vi "MegaAnalysis5.vi"() -> ()   [LabVIEW 2016] (continued)
                            tunnel: w2920 -> [_ _ w2954 w2987]
                            tunnel: [w2924 w2925 w2937 w2970] -> w2919
                            tunnel: [w2924 w2925 w2931 w2964] -> w2918
                            tunnel: [w2924 w2925 w2936 w2969] -> w2917
                            tunnel: [w2924 w2925 w2926 w2959] -> w2916
                            frame 0, Default {
                              w2924 = 0
                            }
                            frame 1 {
                              w2925 = 0
                            }
                            frame 2 {
                              n1178 = call "readbinary.vi"(7:w2956, "base path"=w2954, "file index"=w2955, "data column"="bclr") -> ("data"=w2947:ext[])  [unwired: 7 out]
                              n1179 = call "readbinary.vi"(7:w2956, "base path"=w2954, "file index"=w2955, "data column"="bclf") -> ("data"=w2944:ext[])  [unwired: 7 out]
                              n1180 = Array Max & Min(array=w2944) -> (max value=w2952:ext, min value=w2950:ext)  [unwired: 2 out]
                              n1181 = Array Max & Min(array=w2947) -> (max value=w2953:ext, min value=w2951:ext)  [unwired: 2 out]
                              n1182 = Max & Min(x=w2953, y=w2952) -> (min(x,y)=w2943:ext)  [unwired: 1 out]
                              n1183 = Max & Min(x=w2951, y=w2950) -> (max(x,y)=w2942:ext)  [unwired: 1 out]
                              n1184 = Subtract(x=w2944, y=w2943) -> (x-y=w2941:ext[])
                              n1185 = Subtract(x=w2944, y=w2942) -> (x-y=w2940:ext[])
                              n1186 = Subtract(x=w2947, y=w2943) -> (x-y=w2949:ext[])
                              n1187 = Subtract(x=w2947, y=w2942) -> (x-y=w2946:ext[])
                              n1188 = Absolute Value(x=w2946) -> (abs(x)=w2945:ext[])
                              n1189 = Absolute Value(x=w2941) -> (abs(x)=w2939:ext[])
                              n1190 = Absolute Value(x=w2949) -> (abs(x)=w2948:ext[])
                              n1191 = Absolute Value(x=w2940) -> (abs(x)=w2938:ext[])
                              n1192 = Array Max & Min(array=w2945) -> (min index (indices)=w2934:i32)  [unwired: 3 out]
                              n1193 = Array Max & Min(array=w2948) -> (min index (indices)=w2935:i32)  [unwired: 3 out]
                              n1194 = Array Max & Min(array=w2938) -> (min index (indices)=w2929:i32)  [unwired: 3 out]
                              n1195 = Array Max & Min(array=w2939) -> (min index (indices)=w2930:i32)  [unwired: 3 out]
                              n1196 = Subtract(x=w2935, y=w2934) -> (x-y=w2933:i32)
                              n1197 = Absolute Value(x=w2933) -> (abs(x)=w2932:i32)
                              n1198 = Max & Min(x=w2930, y=w2929) -> (min(x,y)=w2936:i32)  [unwired: 1 out]
                              n1199 = Max & Min(x=w2935, y=w2934) -> (min(x,y)=w2937:i32)  [unwired: 1 out]
                              n1200 = Subtract(x=w2930, y=w2929) -> (x-y=w2928:i32)
                              n1201 = Absolute Value(x=w2928) -> (abs(x)=w2927:i32)
                              n1202 = Increment(x=w2927) -> (x+1=w2926:i32)
                              n1203 = Increment(x=w2932) -> (x+1=w2931:i32)
                            }
                            frame 3 {
                              n1204 = call "readbinary.vi"(7:w2989, "base path"=w2987, "file index"=w2988, "data column"="bclr") -> ("data"=w2980:ext[])  [unwired: 7 out]
                              n1205 = call "readbinary.vi"(7:w2989, "base path"=w2987, "file index"=w2988, "data column"="bclf") -> ("data"=w2977:ext[])  [unwired: 7 out]
                              n1206 = Array Max & Min(array=w2977) -> (max value=w2985:ext, min value=w2983:ext)  [unwired: 2 out]
                              n1207 = Array Max & Min(array=w2980) -> (max value=w2986:ext, min value=w2984:ext)  [unwired: 2 out]
                              n1208 = Max & Min(x=w2986, y=w2985) -> (min(x,y)=w2976:ext)  [unwired: 1 out]
                              n1209 = Max & Min(x=w2984, y=w2983) -> (max(x,y)=w2975:ext)  [unwired: 1 out]
                              n1210 = Subtract(x=w2977, y=w2976) -> (x-y=w2974:ext[])
                              n1211 = Subtract(x=w2977, y=w2975) -> (x-y=w2973:ext[])
                              n1212 = Subtract(x=w2980, y=w2976) -> (x-y=w2982:ext[])
                              n1213 = Subtract(x=w2980, y=w2975) -> (x-y=w2979:ext[])
                              n1214 = Absolute Value(x=w2979) -> (abs(x)=w2978:ext[])
                              n1215 = Absolute Value(x=w2974) -> (abs(x)=w2972:ext[])
                              n1216 = Absolute Value(x=w2982) -> (abs(x)=w2981:ext[])
                              n1217 = Absolute Value(x=w2973) -> (abs(x)=w2971:ext[])
                              n1218 = Array Max & Min(array=w2978) -> (min index (indices)=w2967:i32)  [unwired: 3 out]
                              n1219 = Array Max & Min(array=w2981) -> (min index (indices)=w2968:i32)  [unwired: 3 out]
                              n1220 = Array Max & Min(array=w2971) -> (min index (indices)=w2962:i32)  [unwired: 3 out]
                              n1221 = Array Max & Min(array=w2972) -> (min index (indices)=w2963:i32)  [unwired: 3 out]
                              n1222 = Subtract(x=w2968, y=w2967) -> (x-y=w2966:i32)
                              n1223 = Absolute Value(x=w2966) -> (abs(x)=w2965:i32)
                              n1224 = Max & Min(x=w2963, y=w2962) -> (min(x,y)=w2969:i32)  [unwired: 1 out]
                              n1225 = Max & Min(x=w2968, y=w2967) -> (min(x,y)=w2970:i32)  [unwired: 1 out]
                              n1226 = Subtract(x=w2963, y=w2962) -> (x-y=w2961:i32)
                              n1227 = Absolute Value(x=w2961) -> (abs(x)=w2960:i32)
                              n1228 = Increment(x=w2960) -> (x+1=w2959:i32)
                              n1229 = Increment(x=w2965) -> (x+1=w2964:i32)
                            }
                          }
                        }
                        frame #9 {
                          n1230 = case shown="0, Default" w3001 {
                            tunnel: w3000 -> [_ _ w3010 w3032]
                            tunnel: w2999 -> [_ _ w3009 w3031]
                            tunnel: w2998 -> [_ _ w3008 w3030]
                            tunnel: w2997 -> [_ _ w3007 w3029]
                            tunnel: w2996 -> [_ _ w3006 w3028]
                            tunnel: w2995 -> [_ _ w3005 w3027]
                            tunnel: w2994 -> [_ _ w3004 w3026]
                            tunnel: w2993 -> [_ _ w3003 w3025]
                            tunnel: w2992 -> [_ _ w3002 w3024]
                            frame 0, Default {
                            }
                            frame 1 {
                            }
                            frame 2 {
                              n1231 = for {
                                tunnel: w3010 -> [w3013] mode=indexing
                                tunnel: w3009 -> [w3014] mode=indexing
                                tunnel: w3008 -> [w3012]
                                tunnel: w3007 -> [w3011]
                                tunnel: w3006 -> [w3015]
                                tunnel: w3005 -> [w3021]
                                tunnel: w3004 -> [w3020]
                                tunnel: w3003 -> [w3019]
                                tunnel: w3002 -> [w3018]
                                n1232 = call "readbinary.vi"(7:w3015, "base path"=w3011, "file index"=w3012, "data column"=w3013) -> ("data"=w3023:ext[])  [unwired: 7 out]
                                n1233 = call "readbinary.vi"(7:w3015, "base path"=w3011, "file index"=w3012, "data column"=w3014) -> ("data"=w3022:ext[])  [unwired: 7 out]
                                n1234 = Array Subset(array=w3022, index=w3020, length=w3018) -> (w3016:ext[])
                                n1235 = Array Subset(array=w3023, index=w3021, length=w3019) -> (w3017:ext[])
                                n1236 = call "writebinary.vi"(7:w3015, "base path"=w3011, "file index"=w3012, "data column"=w3014, "data"=w3016) -> ()  [unwired: 7 out]
                                n1237 = call "writebinary.vi"(7:w3015, "base path"=w3011, "file index"=w3012, "data column"=w3013, "data"=w3017) -> ()  [unwired: 7 out]
                              }
                            }
                            frame 3 {
                              n1238 = for {
                                tunnel: w3032 -> [w3035] mode=indexing
                                tunnel: w3031 -> [w3036] mode=indexing
                                tunnel: w3030 -> [w3034]
                                tunnel: w3029 -> [w3033]
                                tunnel: w3028 -> [w3037]
                                tunnel: w3027 -> [w3043]
                                tunnel: w3026 -> [w3042]
                                tunnel: w3025 -> [w3041]
                                tunnel: w3024 -> [w3040]
                                n1239 = call "readbinary.vi"(7:w3037, "base path"=w3033, "file index"=w3034, "data column"=w3035) -> ("data"=w3045:ext[])  [unwired: 7 out]
                                n1240 = call "readbinary.vi"(7:w3037, "base path"=w3033, "file index"=w3034, "data column"=w3036) -> ("data"=w3044:ext[])  [unwired: 7 out]
                                n1241 = Array Subset(array=w3044, index=w3042, length=w3040) -> (w3038:ext[])
                                n1242 = Array Subset(array=w3045, index=w3043, length=w3041) -> (w3039:ext[])
                                n1243 = call "writebinary.vi"(7:w3037, "base path"=w3033, "file index"=w3034, "data column"=w3036, "data"=w3038) -> ()  [unwired: 7 out]
                                n1244 = call "writebinary.vi"(7:w3037, "base path"=w3033, "file index"=w3034, "data column"=w3035, "data"=w3039) -> ()  [unwired: 7 out]
                              }
                            }
                          }
                        }
                      }
                    }
                    n1245 = Boolean To (0,1)(Boolean=w2674) -> (0, 1=w2673:i16[])
                    n1246 = Add Array Elements(numeric array=w2673) -> (sum=w2672:i16)
                    n1247 = Not Equal To 0?(x=w2672) -> (x != 0?=w2669:bool)
                    n1248 = And(x=w2669, y=w2668) -> (x .and. y?=→"dddd":bool)
                  }
                }
              }
            }
          }
          frame #7 {
            n1249 = case shown="True" w3051 {
              tunnel: w3050 -> [_ w3071]
              tunnel: w3049 -> [_ w3072]
              tunnel: w3048 -> [_ w3073]
              tunnel: [w3056 w3062] -> w3047
              tunnel: w3046 -> [_ w3059]
              frame False {
                w3057 = dbl[] [] ("Array 11")
                n1250 = Bundle("Array 11"=w3057, "Array 11"=w3057) -> (w3055:cluster{"Array 11":dbl[], "Array 11":dbl[]})  [unwired: 1 out]
                n1251 = Build Array(w3055) -> (w3056:cluster{"Array 11":dbl[], "Array 11":dbl[]}[])
              }
              frame True {
                n1252 = Build Path(base path=w3071, name or relative path="files2") -> (appended path=w3069:path)
                n1253 = call-poly <vilib>:"Read From Spreadsheet File.vi"("file path (dialog if empty)"=w3069) -> ("first row"=w3060:string[])  [unwired: 3 in, 7 out]
                n1254 = for {
                  tunnel: w3071 -> [w3102]
                  tunnel: w3073 -> [w3106]
                  tunnel: w3072 -> [w3103]
                  tunnel: w3060 -> [_] mode=indexing
                  tunnel: [w3094] -> w3068 mode=indexing
                  tunnel: [w3093] -> w3067 mode=indexing
                  tunnel: w3059 -> [w3092]
                  i -> [w3101]
                  n1255 = Index Array(array=w3106, index="y axis") -> (element=w3099:string)
                  n1256 = Index Array(array=w3103, index="x axis") -> (element=w3098:string)
                  n1257 = Index Array(array=w3106, index="x axis") -> (element=w3097:string)
                  n1258 = Index Array(array=w3103, index="y axis") -> (element=w3100:string)
                  n1259 = call "readbinary.vi"(7:w3092, "base path"=w3102, "file index"=w3101, "data column"=w3098) -> ("data"=w3095:ext[])  [unwired: 7 out]
                  n1260 = call "readbinary.vi"(7:w3092, "base path"=w3102, "file index"=w3101, "data column"=w3097) -> ("data"=w3108:ext[])  [unwired: 7 out]
                  n1261 = call "readbinary.vi"(7:w3092, "base path"=w3102, "file index"=w3101, "data column"=w3099) -> ("data"=w3107:ext[])  [unwired: 7 out]
                  n1262 = call "readbinary.vi"(7:w3092, "base path"=w3102, "file index"=w3101, "data column"=w3100) -> ("data"=w3096:ext[])  [unwired: 7 out]
                  n1263 = Bundle("data"=w3095, "data"=w3096) -> (w3094:cluster{"data":ext[], "data":ext[]})  [unwired: 1 out]
                  n1264 = Bundle("data"=w3108, "data"=w3107) -> (w3093:cluster{"data":ext[], "data":ext[]})  [unwired: 1 out]
                }
                n1265 = Array Size(array=w3060) -> (size(s)=w3066:i32)
                n1266 = Multiply(x=w3066, y=2) -> (x*y=w3064:i32)
                n1267 = global write "status.vi" "String"("plotting selected data") -> ()
                n1268 = for {
                  N: w3064 -> [_]
                  tunnel: w3068 -> [w3076]
                  tunnel: w3067 -> [w3077]
                  shift-right: [w3080] -> _
                  shift-left: 0 -> [w3074]
                  tunnel: [w3075] -> w3062 mode=indexing
                  tunnel: [w3074] -> w3061 mode=indexing
                  i -> [w3078]
                  n1269 = case shown="0, Default" w3074 {
                    tunnel: w3078 -> [w3084 w3091]
                    tunnel: w3077 -> [w3083 _]
                    tunnel: [w3081 w3087] -> w3075
                    tunnel: w3076 -> [_ w3088]
                    frame 0, Default {
                      n1270 = Divide(x=w3084, y=2) -> (x/y=w3082:dbl)
                      n1271 = Index Array(array=w3083, index=w3082) -> (element=w3081:cluster{"data":ext[], "data":ext[]})
                    }
                    frame 1 {
                      n1272 = Decrement(x=w3091) -> (x-1=w3090:i32)
                      n1273 = Divide(x=w3090, y=2) -> (x/y=w3089:dbl)
                      n1274 = Index Array(array=w3088, index=w3089) -> (element=w3087:cluster{"data":ext[], "data":ext[]})
                    }
                  }
                  n1275 = Subtract(x=1, y=w3074) -> (x-y=w3080:i32)
                }
                n1276 = for {
                  tunnel: w3061 -> [_] mode=indexing
                }
              }
            }
            "?" <- w3047
            n1277 = while {
              stop <- w3053 stop-if-true
              n1278 = Not(x="?") -> (.not. x?=w3053:bool)
              n1279 = Wait (ms)(milliseconds to wait=1000) -> ()  [unwired: 1 out]
            }
          }
          frame #8 {
            n1280 = Build Path(base path=w3112, name or relative path="files2") -> (appended path=w3120:path)
            n1281 = Build Path(base path=w3112, name or relative path="paths2") -> (appended path=w3117:path)
            n1282 = call-poly <vilib>:"Read From Spreadsheet File.vi"("file path (dialog if empty)"=w3120) -> ("first row"=w3119:string[])  [unwired: 3 in, 7 out]
            n1283 = call-poly <vilib>:"Read From Spreadsheet File.vi"("file path (dialog if empty)"=w3117) -> ("first row"=w3115:string[])  [unwired: 3 in, 7 out]
            n1284 = String To Path(string=w3115) -> (path=w3116:path[])
            n1285 = case shown="True" w3123 {
              tunnel: w3119 -> [_ w3135]
              tunnel: w3116 -> [_ w3134]
              tunnel: w3122 -> [_ w3133]
              tunnel: w3112 -> [_ w3126]
              tunnel: "file format" -> [_ w3132]
              tunnel: w3113 -> [_ w3131]
              tunnel: w3111 -> [_ w3129]
              tunnel: w3110 -> [w3124 w3128]
              tunnel: [w3124 w3127] -> w3109
              frame False {
              }
              frame True {
                n1286 = for {
                  tunnel: w3135 -> [w3156] mode=indexing
                  tunnel: w3134 -> [w3154] mode=indexing
                  tunnel: "append name" -> [w3155]
                  tunnel: w3133 -> [w3150]
                  tunnel: w3126 -> [w3148]
                  tunnel: w3132 -> [w3145]
                  tunnel: w3131 -> [w3144]
                  tunnel: w3129 -> [w3142]
                  shift-right: [w3140] -> w3127
                  shift-left: w3128 -> [w3139]
                  tunnel: w3126 -> [w3137]
                  i -> [w3149]
                  n1287 = call "filecount.vi"("Path"=w3137) -> ("file count string"=w3136:string)  [unwired: 10 out]
                  n1288 = Concatenate Strings("mega", w3136, w3156, w3155) -> (w3153:string)
                  n1289 = Build Path(base path=w3154, name or relative path=w3153) -> (appended path=w3138:path)
                  n1290 = Build Array (concatenate)(w3138, w3139) -> (w3140:path[])
                  n1291 = Array Size(array=w3150) -> (size(s)=w3152:i32)
                  n1292 = Decrement(x=w3152) -> (x-1=w3151:i32)
                  n1293 = for {
                    N: w3151 -> [_]
                    tunnel: w3150 -> [w3178]
                    tunnel: w3149 -> [w3173]
                    tunnel: w3148 -> [w3172]
                    tunnel: [w3168] -> w3146 mode=indexing
                    tunnel: w3144 -> [w3176]
                    tunnel: "saving order" -> [w3171]
                    tunnel: w3142 -> [w3167]
                    i -> [w3179]
                    n1294 = Increment(x=w3179) -> (x+1=w3175:i32)
                    n1295 = Index Array(array=w3176, index=w3175) -> (element=w3174:string)
                    n1296 = Index Array(array=w3178, index=w3175) -> (element=w3177:string)
                    n1297 = call "readbinary.vi"(7:w3167, "base path"=w3172, "file index"=w3173, "data column"=w3174) -> ("data"=w3170:ext[])  [unwired: 7 out]
                    n1298 = call "readbinary.vi"(7:w3167, "base path"=w3172, "file index"=w3173, "data column"=w3177) -> ("data"=w3169:ext[])  [unwired: 7 out]
                    n1299 = case shown="1" w3171 {
                      tunnel: w3170 -> [w3181 w3185]
                      tunnel: w3169 -> [w3180 w3184]
                      tunnel: [w3182 w3183] -> w3168
                      frame 0, Default {
                        n1300 = Build Array (concatenate)(w3180, w3181) -> (w3182:ext[])
                      }
                      frame 1 {
                        n1301 = Build Array (concatenate)(w3185, w3184) -> (w3183:ext[])
                      }
                    }
                  }
                  n1302 = stacked-sequence {
                    tunnel: "time\tdB/dt\tBfield\tdata\n" -> [_ w3162 _]
                    tunnel: w3138 -> [w3157 w3161 w3165]
                    tunnel: w3146 -> [_ _ w3166]
                    tunnel: w3145 -> [_ _ w3164]
                    frame #0 {
                      n1303 = call <vilib>:"Check if File or Folder Exists.vi"("path"=w3157) -> ("file or folder exists?"=w3158:bool)  [unwired: 1 in, 9 out]
                      n1304 = case shown="True" w3158 {
                        selector: w3158 -> [_ w3160]
                        tunnel: w3157 -> [_ w3159]
                        frame False {
                        }
                        frame True {
                          n1305 = Delete(path (use dialog)=w3159, entire hierarchy (F)=w3160) -> ()  [unwired: 1 in, 5 out]
                        }
                      }
                    }
                    frame #1 {
                      n1306 = Write to Text File(file (use dialog)=w3161, text=w3162) -> ()  [unwired: 1 in, 4 out]
                    }
                    frame #2 {
                      w3163 = TRUE
                      n1307 = call "Write To Spreadsheet File2.vi"("transpose? (no:F)"=w3163, "format (%d)"=w3164, "append to file? (new file:F)"=w3163, "2D data"=w3166, "file path (dialog if empty)"=w3165) -> ()  [unwired: 3 in, 1 out]
                    }
                  }
                }
                n1308 = global write "status.vi" "String"("saving selected data") -> ()
              }
            }
          }
          frame #9 {
            w3188 = FALSE  # Set axes names
            n1309 = Build Path(base path=w3202, name or relative path="files2") -> (appended path=w3200:path)
            n1310 = call-poly <vilib>:"Read From Spreadsheet File.vi"("file path (dialog if empty)"=w3200) -> ("first row"=w3191:string[])  [unwired: 3 in, 7 out]
            n1311 = case shown="0, Default" "label" {
              tunnel: w3191 -> [w3210 _ _]
              tunnel: [w3209 w3221 w3232] -> w3198
              tunnel: [w3208 w3220 w3231] -> w3197
              frame 0, Default {
                n1312 = for {
                  tunnel: w3210 -> [w3215] mode=indexing
                  tunnel: [w3214] -> w3209 mode=indexing
                  tunnel: [w3213] -> w3208 mode=indexing
                  n1313 = Concatenate Strings("falling_", w3215) -> (w3213:string)
                  n1314 = Concatenate Strings("rising_", w3215) -> (w3214:string)
                }
              }
              frame 1 {
                n1315 = property on="angle theta (cos theta renorm.)" class="Arr (strict)"() -> ("Value"=w3219:ext[])  [unwired: 2 in, 2 out]
                n1316 = Number To Fractional String(number=w3219, width (-)=10, precision (6)=3) -> (F-format string=w3218:string[])  [unwired: 1 out]
                n1317 = for {
                  tunnel: w3218 -> [w3226] mode=indexing
                  tunnel: [w3225] -> w3221 mode=indexing
                  tunnel: [w3224] -> w3220 mode=indexing
                  n1318 = Concatenate Strings("falling:", w3226) -> (w3224:string)
                  n1319 = Concatenate Strings("rising:", w3226) -> (w3225:string)
                }
              }
              frame 2 {
                n1320 = property on="variable (T)" class="Arr (strict)"() -> ("Value"=w3229:dbl[])  [unwired: 2 in, 2 out]
                n1321 = Number To Fractional String(number=w3229, width (-)=10, precision (6)=3) -> (F-format string=w3230:string[])  [unwired: 1 out]
                n1322 = for {
                  tunnel: w3230 -> [w3237] mode=indexing
                  tunnel: [w3236] -> w3232 mode=indexing
                  tunnel: [w3235] -> w3231 mode=indexing
                  n1323 = Concatenate Strings("falling:", w3237) -> (w3235:string)
                  n1324 = Concatenate Strings("rising:", w3237) -> (w3236:string)
                }
              }
            }
            n1325 = for {
              tunnel: [w3203] -> w3195 mode=indexing
              tunnel: w3191 -> [_] mode=indexing
              i -> [w3203]
            }
            n1326 = Number To Decimal String(number=w3195, width (-)=3) -> (decimal integer string=w3193:string[])
            n1327 = Build Array(w3193, w3191) -> (w3192:string[][])
            n1328 = Transpose 2D Array(2D array=w3192) -> (transposed array=→"file list":string[][])
            n1329 = for {
              tunnel: w3198 -> [w3207] mode=indexing
              tunnel: w3197 -> [w3205] mode=indexing
              shift-right: [w3204] -> w3187
              shift-left: string[] [] ("Array 26") -> [w3206]
              n1330 = Build Array (concatenate)(w3206, w3207, w3205) -> (w3204:string[])
            }
            n1331 = control-ref of="?"() -> (w3189:refnum<vi>)
            n1332 = call "Neilsetplot.vi"("Set axes names"=w3188, "max # rows (-1:all)"=-1, "Plot names"=w3187, "XYGraph Refnum"=w3189) -> ()  [unwired: 6 in, 2 out]
          }
        }
      }
      frame #6 {
        # "interp frame"
        n1333 = Or(x=w3240, y="?") -> (x .or. y?=w3242:bool)
        n1334 = stacked-sequence {
          tunnel: w3242 -> [_ w3299 w4063 w4323 w4388 _ _]
          tunnel: w3251 -> [w3257 w3298 w4069 w4316 w4395 w4480 w4567]
          tunnel: "?" -> [_ _ w4072 _ _ w4473 _]
          tunnel: w3249 -> [_ _ w4074 _ _ w4472 _]
          tunnel: "?" -> [_ _ w4070 _ _ _ _]
          tunnel: w3246 -> [_ _ w4068 _ _ _ _]
          tunnel: "x axis" -> [_ _ _ w4313 _ w4470 _]
          tunnel: w3245 -> [w3252 w3297 w4062 w4312 w4387 w4469 w4566]
          tunnel: w3244 -> [_ w3296 _ _ _ _ _]
          tunnel: w3243 -> [w3253 _ _ _ _ _ _]
          tunnel: w3239 -> [_ _ _ _ _ _ w4565]
          tunnel: [_ _ _ _ _ _ w4564] -> w3238
          frame #0 {
            n1335 = Build Array("timi", "bdti", "bcli", "dati", "temp", "hold") -> (w3256:string[])
            n1336 = Build Path(base path=w3257, name or relative path="files2") -> (appended path=w3259:path)
            n1337 = call-poly <vilib>:"Read From Spreadsheet File.vi"("file path (dialog if empty)"=w3259) -> ("first row"=w3258:string[])  [unwired: 3 in, 7 out]
            n1338 = stacked-sequence {
              tunnel: w3258 -> [w3267 w3277]
              tunnel: w3257 -> [w3266 w3279]
              tunnel: w3256 -> [w3265 w3278]
              tunnel: w3253 -> [_ w3275]
              tunnel: w3252 -> [_ w3274]
              frame #0 {
                n1339 = for {
                  tunnel: w3265 -> [w3270]
                  tunnel: w3266 -> [w3269]
                  tunnel: w3267 -> [_] mode=indexing
                  i -> [w3268]
                  n1340 = for {
                    tunnel: w3270 -> [w3273] mode=indexing
                    tunnel: w3269 -> [w3272]
                    tunnel: w3268 -> [w3271]
                    n1341 = call "createemptybinary.vi"("base path"=w3272, "file index"=w3271, "data column"=w3273) -> ()  [unwired: 9 out]
                  }
                }
              }
              frame #1 {
                n1342 = Equal?(x=w3275, y=w3274) -> (x = y?=w3276:bool)
                n1343 = case shown="True" w3276 {
                  tunnel: w3277 -> [w3284 _]
                  tunnel: w3278 -> [w3283 _]
                  tunnel: w3279 -> [w3282 _]
                  tunnel: w3275 -> [w3281 _]
                  tunnel: w3274 -> [w3280 _]
                  frame False {
                    n1344 = for {
                      tunnel: w3284 -> [_] mode=indexing
                      tunnel: w3283 -> [w3289]
                      tunnel: w3282 -> [w3287]
                      tunnel: w3281 -> [w3286]
                      tunnel: w3280 -> [w3285]
                      i -> [w3288]
                      n1345 = for {
                        tunnel: w3289 -> [w3292] mode=indexing
                        tunnel: w3288 -> [w3291]
                        tunnel: w3287 -> [w3290]
                        tunnel: w3286 -> [w3295]
                        tunnel: w3285 -> [w3293]
                        n1346 = call "readbinary.vi"(7:w3295, "base path"=w3290, "file index"=w3291, "data column"=w3292) -> ("data"=w3294:ext[])  [unwired: 7 out]
                        n1347 = call "writebinary.vi"(7:w3293, "base path"=w3290, "file index"=w3291, "data column"=w3292, "data"=w3294) -> ()  [unwired: 7 out]
                      }
                    }
                  }
                  frame True {
                  }
                }
              }
            }
          }
          frame #1 {
            n1348 = case shown="True" w3299 {
              tunnel: w3298 -> [w3300 w3308]
              tunnel: w3297 -> [_ w3306]
              tunnel: w3296 -> [_ w3305]
              frame False {
                n1349 = call "createemptybinary.vi"("base path"=w3300, "file index"=0, "data column"="inte") -> ()  [unwired: 9 out]
              }
              frame True {
                n1350 = stacked-sequence {
                  seq-local: [w3310 _ _ _ _ _ _ _] -> [_ w3329 w3363 w3796 w3806 w3925 w3991 _]
                  seq-local: [_ w3335 _ _ _ _ _ _] -> [_ _ w3352 _ _ _ _ _]
                  seq-local: [_ _ "interpolate in:" _ _ _ _ _] -> [_ _ _ w3795 _ _ _ _]
                  seq-local: [w3311 _ _ _ _ _ _ _] -> [_ _ w3358 _ _ _ _ _]
                  seq-local: [_ w3331 _ _ _ _ _ _] -> [_ _ w3355 _ _ _ _ _]
                  seq-local: [_ w3330 _ _ _ _ _ _] -> [_ _ w3354 _ _ _ _ _]
                  seq-local: [_ _ _ _ _ w3918 _ _] -> [_ _ _ _ _ _ w3988 _]
                  tunnel: w3308 -> [w3316 _ w3360 w3793 w3807 w3921 w3990 _]
                  tunnel: "rising and falling field options" -> [_ _ w3361 _ _ _ _ _]
                  tunnel: w3306 -> [_ _ w3356 w3790 w3805 w3919 w3989 _]
                  tunnel: w3305 -> [w3309 _ w3357 _ _ _ _ _]
                  tunnel: "?" -> [_ _ w3353 _ _ _ _ _]
                  frame #0 {
                    w3317 = 0
                    n1351 = Build Path(base path=w3316, name or relative path="paths2") -> (appended path=w3325:path)
                    n1352 = Build Path(base path=w3316, name or relative path="files2") -> (appended path=w3326:path)
                    n1353 = call "readbinary.vi"(7:w3309, "base path"=w3316, "file index"=w3317, "data column"="indf") -> ("data"=w3314:ext[])  [unwired: 7 out]
                    n1354 = call "readbinary.vi"(7:w3309, "base path"=w3316, "file index"=w3317, "data column"="indr") -> ("data"=w3315:ext[])  [unwired: 7 out]
                    n1355 = call-poly <vilib>:"Read From Spreadsheet File.vi"("file path (dialog if empty)"=w3325) -> ("first row"=w3320:string[])  [unwired: 3 in, 7 out]
                    n1356 = call-poly <vilib>:"Read From Spreadsheet File.vi"("file path (dialog if empty)"=w3326) -> ("first row"=w3310:string[])  [unwired: 3 in, 7 out]
                    n1357 = Array Size(array=w3314) -> (size(s)=w3312:i32)
                    n1358 = Array Size(array=w3315) -> (size(s)=w3313:i32)
                    n1359 = Greater?(x=w3313, y=w3312) -> (0:w3311:bool)
                    n1360 = Build Path(base path=w3316, name or relative path="files3") -> (appended path=w3322:path)
                    n1361 = Build Path(base path=w3316, name or relative path="paths3") -> (appended path=w3321:path)
                    n1362 = call-poly <vilib>:"Write To Spreadsheet File.vi"("1D data"=w3310, "file path (dialog if empty)"=w3322) -> ()  [unwired: 4 in, 3 out]
                    n1363 = call-poly <vilib>:"Write To Spreadsheet File.vi"("1D data"=w3320, "file path (dialog if empty)"=w3321) -> ()  [unwired: 4 in, 3 out]
                  }
                  frame #1 {
                    n1364 = property class="Bool (strict)"() -> ("Value"=w3334:bool)  [unwired: 2 in, 2 out]
                    n1365 = property class="Arr (strict)"() -> ("Value"=w3333:cluster{dbl, "and":dbl}[])  [unwired: 2 in, 2 out]
                    n1366 = Decrement(x="# points") -> (x-1=w3336:u64)
                    n1367 = for {
                      N: "# points" -> [_]
                      tunnel: [w3351] -> w3337 mode=indexing
                      i -> [w3351]
                    }
                    n1368 = case shown="True" w3334 {
                      tunnel: w3333 -> [w3344 w3347]
                      tunnel: [w3344 w3346] -> w3332
                      tunnel: w3329 -> [_ w3345]
                      frame False {
                      }
                      frame True {
                        n1369 = for {
                          tunnel: w3347 -> [w3350]
                          tunnel: [w3348] -> w3346 mode=indexing
                          tunnel: w3345 -> [_] mode=indexing
                          n1370 = Index Array(array=w3350, index=0) -> (element=w3348:cluster{dbl, "and":dbl})
                        }
                      }
                    }
                    n1371 = Divide(x=w3337, y=w3336) -> (x/y=w3335:dbl[])
                    n1372 = for {
                      tunnel: w3332 -> [w3343] mode=indexing
                      tunnel: [w3340] -> w3331 mode=indexing
                      tunnel: [w3339] -> w3330 mode=indexing
                      n1373 = Unbundle(w3343) -> (w3342:dbl, "and"=w3341:dbl)
                      n1374 = Max & Min(x=w3342, y=w3341) -> (max(x,y)=w3339:dbl, min(x,y)=w3340:dbl)
                    }
                  }
                  frame #2 {
                    n1375 = for {
                      tunnel: w3363 -> [_] mode=indexing
                      tunnel: "interpolate in:" -> [w3384]
                      tunnel: w3360 -> [w3382]
                      tunnel: w3352 -> [w3383]
                      tunnel: "method" -> [w3381]
                      tunnel: w3361 -> [w3380]
                      tunnel: w3360 -> [w3374]
                      tunnel: w3358 -> [w3369]
                      tunnel: w3357 -> [w3368]
                      tunnel: w3356 -> [w3364]
                      tunnel: w3355 -> [w3367] mode=indexing
                      tunnel: w3354 -> [w3366] mode=indexing
                      tunnel: w3353 -> [w3365]
                      i -> [w3375]
                      n1376 = case shown="3" w3384 {
                        tunnel: w3382 -> [w3543 w3609 w3687 w3760]
                        tunnel: w3375 -> [w3542 w3608 w3686 w3759]
                        tunnel: w3383 -> [w3531 w3603 w3680 w3750]
                        tunnel: w3381 -> [w3528 w3600 w3678 w3747]
                        tunnel: [w3525 w3584 w3662 w3735] -> w3379
                        tunnel: [w3524 w3583 w3661 w3734] -> w3373
                        tunnel: [w3523 w3597 w3675 w3744] -> w3378
                        tunnel: [w3522 w3596 w3674 w3743] -> w3372
                        tunnel: [w3521 w3586 w3660 w3729] -> w3377
                        tunnel: [w3520 w3585 w3659 w3728] -> w3371
                        tunnel: [w3519 w3595 w3673 w3731] -> w3376
                        tunnel: [w3518 w3594 w3672 w3730] -> w3370
                        tunnel: w3368 -> [w3510 w3582 w3658 w3727]
                        tunnel: w3367 -> [_ w3577 w3652 _]
                        tunnel: w3366 -> [_ w3576 w3651 _]
                        tunnel: w3365 -> [_ w3575 w3650 _]
                        frame 0, Default {
                          n1377 = Build Array("bdti", "bcli", "dati") -> (w3553:string[])
                          n1378 = Build Array("bdtr", "bclr", "datr") -> (w3546:string[])
                          n1379 = Build Array("bdtf", "bclf", "datf") -> (w3545:string[])
                          n1380 = call "readbinary.vi"(7:w3510, "base path"=w3543, "file index"=w3542, "data column"="timr") -> ("data"=w3541:ext[])  [unwired: 7 out]
                          n1381 = call "readbinary.vi"(7:w3510, "base path"=w3543, "file index"=w3542, "data column"="timf") -> ("data"=w3533:ext[])  [unwired: 7 out]
                          n1382 = Array Max & Min(array=w3541) -> (max value=w3540:ext, min value=w3537:ext)  [unwired: 2 out]
                          n1383 = Array Max & Min(array=w3533) -> (max value=w3532:ext, min value=w3534:ext)  [unwired: 2 out]
                          n1384 = Subtract(x=w3540, y=w3537) -> (x-y=w3539:ext)
                          n1385 = Subtract(x=w3532, y=w3534) -> (x-y=w3536:ext)
                          n1386 = Multiply(x=w3531, y=w3539) -> (x*y=w3538:ext[])
                          n1387 = Multiply(x=w3531, y=w3536) -> (x*y=w3535:ext[])
                          n1388 = Add(x=w3538, y=w3537) -> (x+y=w3529:ext[])
                          n1389 = Add(x=w3535, y=w3534) -> (x+y=w3530:ext[])
                          n1390 = for {
                            tunnel: w3553 -> [_] mode=indexing
                            tunnel: w3546 -> [w3571] mode=indexing
                            tunnel: w3545 -> [w3572] mode=indexing
                            tunnel: w3543 -> [w3570]
                            tunnel: w3542 -> [w3569]
                            tunnel: w3541 -> [w3568]
                            tunnel: w3533 -> [w3567]
                            tunnel: w3530 -> [w3564]
                            tunnel: w3529 -> [w3563]
                            tunnel: w3528 -> [w3562]
                            tunnel: [w3561] -> w3527 mode=indexing
                            tunnel: [w3560] -> w3525
                            tunnel: [w3559] -> w3526 mode=indexing
                            tunnel: [w3558] -> w3524
                            tunnel: w3510 -> [w3557]
                            n1391 = call "readbinary.vi"(7:w3557, "base path"=w3570, "file index"=w3569, "data column"=w3571) -> ("data"=w3566:ext[])  [unwired: 7 out]
                            n1392 = call "readbinary.vi"(7:w3557, "base path"=w3570, "file index"=w3569, "data column"=w3572) -> ("data"=w3565:ext[])  [unwired: 7 out]
                            n1393 = call <vilib>:"Interpolate 1D.vi"("method"=w3562, "xi"=w3563, "X"=w3568, "Y"=w3566) -> ("xi used"=w3560:dbl[], "yi"=w3561:dbl[])  [unwired: 2 in, 4 out]
                            n1394 = call <vilib>:"Interpolate 1D.vi"("method"=w3562, "xi"=w3564, "X"=w3567, "Y"=w3565) -> ("xi used"=w3558:dbl[], "yi"=w3559:dbl[])  [unwired: 2 in, 4 out]
                          }
                          n1395 = Index Array(array=w3527, index (row)=0) -> (element=w3523:dbl[])  [unwired: 1 in]
                          n1396 = Index Array(array=w3527, index (row)=1) -> (element=w3521:dbl[])  [unwired: 1 in]
                          n1397 = Index Array(array=w3527, index (row)=2) -> (element=w3519:dbl[])  [unwired: 1 in]
                          n1398 = Index Array(array=w3526, index (row)=0) -> (element=w3522:dbl[])  [unwired: 1 in]
                          n1399 = Index Array(array=w3526, index (row)=1) -> (element=w3520:dbl[])  [unwired: 1 in]
                          n1400 = Index Array(array=w3526, index (row)=2) -> (element=w3518:dbl[])  [unwired: 1 in]
                        }
                        frame 1 {
                          n1401 = Build Array("bdti", "timi", "dati") -> (w3619:string[])
                          n1402 = Build Array("bdtr", "timr", "datr") -> (w3612:string[])
                          n1403 = Build Array("bdtf", "timf", "datf") -> (w3611:string[])
                          n1404 = call "readbinary.vi"(7:w3582, "base path"=w3609, "file index"=w3608, "data column"="bclr") -> ("data"=w3573:ext[])  [unwired: 7 out]
                          n1405 = call "readbinary.vi"(7:w3582, "base path"=w3609, "file index"=w3608, "data column"="bclf") -> ("data"=w3574:ext[])  [unwired: 7 out]
                          n1406 = case shown="True" w3575 {
                            tunnel: [w3624 w3630] -> w3581
                            tunnel: [w3623 w3629] -> w3580
                            tunnel: [w3624 w3628] -> w3579
                            tunnel: [w3623 w3627] -> w3578
                            tunnel: w3573 -> [_ w3626]
                            tunnel: w3574 -> [_ w3625]
                            tunnel: w3577 -> [w3624 _]
                            tunnel: w3576 -> [w3623 _]
                            frame False {
                            }
                            frame True {
                              n1407 = Array Max & Min(array=w3626) -> (max value=w3630:ext, min value=w3629:ext)  [unwired: 2 out]
                              n1408 = Array Max & Min(array=w3625) -> (max value=w3628:ext, min value=w3627:ext)  [unwired: 2 out]
                            }
                          }
                          n1409 = Subtract(x=w3581, y=w3580) -> (x-y=w3607:ext)
                          n1410 = Subtract(x=w3579, y=w3578) -> (x-y=w3605:ext)
                          n1411 = Multiply(x=w3603, y=w3607) -> (x*y=w3606:ext[])
                          n1412 = Multiply(x=w3603, y=w3605) -> (x*y=w3604:ext[])
                          n1413 = Add(x=w3604, y=w3578) -> (x+y=w3602:ext[])
                          n1414 = Add(x=w3606, y=w3580) -> (x+y=w3601:ext[])
                          n1415 = for {
                            tunnel: w3619 -> [_] mode=indexing
                            tunnel: w3612 -> [w3645] mode=indexing
                            tunnel: w3611 -> [w3646] mode=indexing
                            tunnel: w3609 -> [w3644]
                            tunnel: w3608 -> [w3643]
                            tunnel: w3573 -> [w3642]
                            tunnel: w3574 -> [w3641]
                            tunnel: w3602 -> [w3638]
                            tunnel: w3601 -> [w3637]
                            tunnel: w3600 -> [w3636]
                            tunnel: [w3635] -> w3599 mode=indexing
                            tunnel: [w3634] -> w3586
                            tunnel: [w3633] -> w3598 mode=indexing
                            tunnel: [w3632] -> w3585
                            tunnel: w3582 -> [w3631]
                            n1416 = call "readbinary.vi"(7:w3631, "base path"=w3644, "file index"=w3643, "data column"=w3645) -> ("data"=w3640:ext[])  [unwired: 7 out]
                            n1417 = call "readbinary.vi"(7:w3631, "base path"=w3644, "file index"=w3643, "data column"=w3646) -> ("data"=w3639:ext[])  [unwired: 7 out]
                            n1418 = call <vilib>:"Interpolate 1D.vi"("method"=w3636, "xi"=w3637, "X"=w3642, "Y"=w3640) -> ("xi used"=w3634:dbl[], "yi"=w3635:dbl[])  [unwired: 2 in, 4 out]
                            n1419 = call <vilib>:"Interpolate 1D.vi"("method"=w3636, "xi"=w3638, "X"=w3641, "Y"=w3639) -> ("xi used"=w3632:dbl[], "yi"=w3633:dbl[])  [unwired: 2 in, 4 out]
                          }
                          n1420 = Index Array(array=w3599, index (row)=0) -> (element=w3597:dbl[])  [unwired: 1 in]
                          n1421 = Index Array(array=w3599, index (row)=1) -> (element=w3584:dbl[])  [unwired: 1 in]
                          n1422 = Index Array(array=w3599, index (row)=2) -> (element=w3595:dbl[])  [unwired: 1 in]
                          n1423 = Index Array(array=w3598, index (row)=0) -> (element=w3596:dbl[])  [unwired: 1 in]
                          n1424 = Index Array(array=w3598, index (row)=1) -> (element=w3583:dbl[])  [unwired: 1 in]
                          n1425 = Index Array(array=w3598, index (row)=2) -> (element=w3594:dbl[])  [unwired: 1 in]
                        }
                        frame 2 {
                          n1426 = Build Array("bdti", "timi", "dati") -> (w3697:string[])
                          n1427 = Build Array("bdtr", "timr", "datr") -> (w3690:string[])
                          n1428 = Build Array("bdtf", "timf", "datf") -> (w3689:string[])
                          n1429 = call "readbinary.vi"(7:w3658, "base path"=w3687, "file index"=w3686, "data column"="bclf") -> ("data"=w3681:ext[])  [unwired: 7 out]
                          n1430 = call "readbinary.vi"(7:w3658, "base path"=w3687, "file index"=w3686, "data column"="bclr") -> ("data"=w3685:ext[])  [unwired: 7 out]
                          n1431 = Reciprocal(x=w3685) -> (1/x=w3654:ext[])
                          n1432 = Reciprocal(x=w3681) -> (1/x=w3653:ext[])
                          n1433 = case shown="False" w3650 {
                            tunnel: [w3702 w3710] -> w3657
                            tunnel: [w3703 w3709] -> w3656
                            tunnel: [w3702 w3708] -> w3655
                            tunnel: [w3703 w3707] -> w3649
                            tunnel: w3652 -> [w3704 _]
                            tunnel: w3651 -> [w3701 _]
                            tunnel: w3654 -> [_ w3706]
                            tunnel: w3653 -> [_ w3705]
                            frame False {
                              n1434 = Reciprocal(x=w3704) -> (1/x=w3703:dbl)
                              n1435 = Reciprocal(x=w3701) -> (1/x=w3702:dbl)
                            }
                            frame True {
                              n1436 = Array Max & Min(array=w3706) -> (max value=w3710:ext, min value=w3709:ext)  [unwired: 2 out]
                              n1437 = Array Max & Min(array=w3705) -> (max value=w3708:ext, min value=w3707:ext)  [unwired: 2 out]
                            }
                          }
                          n1438 = Subtract(x=w3655, y=w3649) -> (x-y=w3648:ext)
                          n1439 = Subtract(x=w3657, y=w3656) -> (x-y=w3684:ext)
                          n1440 = Multiply(x=w3680, y=w3684) -> (x*y=w3683:ext[])
                          n1441 = Multiply(x=w3680, y=w3648) -> (x*y=w3682:ext[])
                          n1442 = Add(x=w3682, y=w3649) -> (x+y=w3679:ext[])
                          n1443 = Add(x=w3683, y=w3656) -> (x+y=w3647:ext[])
                          n1444 = for {
                            tunnel: w3697 -> [_] mode=indexing
                            tunnel: w3690 -> [w3725] mode=indexing
                            tunnel: w3689 -> [w3726] mode=indexing
                            tunnel: w3687 -> [w3724]
                            tunnel: w3686 -> [w3723]
                            tunnel: w3654 -> [w3722]
                            tunnel: w3653 -> [w3721]
                            tunnel: w3679 -> [w3718]
                            tunnel: w3647 -> [w3717]
                            tunnel: w3678 -> [w3716]
                            tunnel: [w3715] -> w3677 mode=indexing
                            tunnel: [w3714] -> w3664
                            tunnel: [w3713] -> w3676 mode=indexing
                            tunnel: [w3712] -> w3663
                            tunnel: w3658 -> [w3711]
                            n1445 = call "readbinary.vi"(7:w3711, "base path"=w3724, "file index"=w3723, "data column"=w3725) -> ("data"=w3720:ext[])  [unwired: 7 out]
                            n1446 = call "readbinary.vi"(7:w3711, "base path"=w3724, "file index"=w3723, "data column"=w3726) -> ("data"=w3719:ext[])  [unwired: 7 out]
                            n1447 = call <vilib>:"Interpolate 1D.vi"("method"=w3716, "xi"=w3717, "X"=w3722, "Y"=w3720) -> ("xi used"=w3714:dbl[], "yi"=w3715:dbl[])  [unwired: 2 in, 4 out]
                            n1448 = call <vilib>:"Interpolate 1D.vi"("method"=w3716, "xi"=w3718, "X"=w3721, "Y"=w3719) -> ("xi used"=w3712:dbl[], "yi"=w3713:dbl[])  [unwired: 2 in, 4 out]
                          }
                          n1449 = Index Array(array=w3677, index (row)=0) -> (element=w3675:dbl[])  [unwired: 1 in]
                          n1450 = Index Array(array=w3677, index (row)=1) -> (element=w3662:dbl[])  [unwired: 1 in]
                          n1451 = Index Array(array=w3677, index (row)=2) -> (element=w3673:dbl[])  [unwired: 1 in]
                          n1452 = Reciprocal(x=w3664) -> (1/x=w3660:dbl[])
                          n1453 = Reciprocal(x=w3663) -> (1/x=w3659:dbl[])
                          n1454 = Index Array(array=w3676, index (row)=0) -> (element=w3674:dbl[])  [unwired: 1 in]
                          n1455 = Index Array(array=w3676, index (row)=1) -> (element=w3661:dbl[])  [unwired: 1 in]
                          n1456 = Index Array(array=w3676, index (row)=2) -> (element=w3672:dbl[])  [unwired: 1 in]
                        }
                        frame 3 {
                          n1457 = Build Array("bdti", "timi", "bcli") -> (w3770:string[])
                          n1458 = Build Array("bdtr", "timr", "bclr") -> (w3763:string[])
                          n1459 = Build Array("bdtf", "timf", "bclf") -> (w3762:string[])
                          n1460 = call "readbinary.vi"(7:w3727, "base path"=w3760, "file index"=w3759, "data column"="datf") -> ("data"=w3732:ext[])  [unwired: 7 out]
                          n1461 = call "readbinary.vi"(7:w3727, "base path"=w3760, "file index"=w3759, "data column"="datr") -> ("data"=w3733:ext[])  [unwired: 7 out]
                          n1462 = Array Max & Min(array=w3733) -> (max value=w3758:ext, min value=w3755:ext)  [unwired: 2 out]
                          n1463 = Array Max & Min(array=w3732) -> (max value=w3751:ext, min value=w3752:ext)  [unwired: 2 out]
                          n1464 = Subtract(x=w3758, y=w3755) -> (x-y=w3757:ext)
                          n1465 = Subtract(x=w3751, y=w3752) -> (x-y=w3754:ext)
                          n1466 = Multiply(x=w3750, y=w3754) -> (x*y=w3753:ext[])
                          n1467 = Multiply(x=w3750, y=w3757) -> (x*y=w3756:ext[])
                          n1468 = Add(x=w3753, y=w3752) -> (x+y=w3749:ext[])
                          n1469 = Add(x=w3756, y=w3755) -> (x+y=w3748:ext[])
                          n1470 = for {
                            tunnel: w3770 -> [_] mode=indexing
                            tunnel: w3763 -> [w3788] mode=indexing
                            tunnel: w3762 -> [w3789] mode=indexing
                            tunnel: w3760 -> [w3787]
                            tunnel: w3759 -> [w3786]
                            tunnel: w3733 -> [w3785]
                            tunnel: w3732 -> [w3784]
                            tunnel: w3749 -> [w3781]
                            tunnel: w3748 -> [w3780]
                            tunnel: w3747 -> [w3779]
                            tunnel: [w3778] -> w3746 mode=indexing
                            tunnel: [w3777] -> w3731
                            tunnel: [w3776] -> w3745 mode=indexing
                            tunnel: [w3775] -> w3730
                            tunnel: w3727 -> [w3774]
                            n1471 = call "readbinary.vi"(7:w3774, "base path"=w3787, "file index"=w3786, "data column"=w3788) -> ("data"=w3783:ext[])  [unwired: 7 out]
                            n1472 = call "readbinary.vi"(7:w3774, "base path"=w3787, "file index"=w3786, "data column"=w3789) -> ("data"=w3782:ext[])  [unwired: 7 out]
                            n1473 = call <vilib>:"Interpolate 1D.vi"("method"=w3779, "xi"=w3780, "X"=w3785, "Y"=w3783) -> ("xi used"=w3777:dbl[], "yi"=w3778:dbl[])  [unwired: 2 in, 4 out]
                            n1474 = call <vilib>:"Interpolate 1D.vi"("method"=w3779, "xi"=w3781, "X"=w3784, "Y"=w3782) -> ("xi used"=w3775:dbl[], "yi"=w3776:dbl[])  [unwired: 2 in, 4 out]
                          }
                          n1475 = Index Array(array=w3746, index (row)=0) -> (element=w3744:dbl[])  [unwired: 1 in]
                          n1476 = Index Array(array=w3746, index (row)=1) -> (element=w3735:dbl[])  [unwired: 1 in]
                          n1477 = Index Array(array=w3746, index (row)=2) -> (element=w3729:dbl[])  [unwired: 1 in]
                          n1478 = Index Array(array=w3745, index (row)=0) -> (element=w3743:dbl[])  [unwired: 1 in]
                          n1479 = Index Array(array=w3745, index (row)=1) -> (element=w3734:dbl[])  [unwired: 1 in]
                          n1480 = Index Array(array=w3745, index (row)=2) -> (element=w3728:dbl[])  [unwired: 1 in]
                        }
                      }
                      n1481 = case shown="2" w3380 {
                        tunnel: w3379 -> [w3395 _ w3424 w3449 w3474 w3494]
                        tunnel: w3378 -> [w3394 _ w3420 w3445 w3470 w3492]
                        tunnel: w3377 -> [w3393 _ w3415 w3440 w3465 w3490]
                        tunnel: w3376 -> [w3392 _ w3410 w3435 w3458 w3488]
                        tunnel: w3375 -> [w3387 w3402 w3427 w3452 w3477 w3497]
                        tunnel: w3374 -> [w3386 w3401 w3426 w3451 w3476 w3496]
                        tunnel: w3373 -> [_ w3400 w3425 w3450 w3475 w3493]
                        tunnel: w3372 -> [_ w3399 w3419 w3444 w3469 w3491]
                        tunnel: w3371 -> [_ w3398 w3414 w3439 w3464 w3489]
                        tunnel: w3370 -> [_ w3397 w3409 w3434 w3459 w3487]
                        tunnel: w3369 -> [_ _ _ _ _ w3495]
                        tunnel: w3364 -> [w3385 w3396 w3407 w3432 w3457 w3482]
                        frame 0, Default {
                          n1482 = call "writebinary.vi"(7:w3385, "base path"=w3386, "file index"=w3387, "data column"="dati", "data"=w3392) -> ()  [unwired: 7 out]
                          n1483 = call "writebinary.vi"(7:w3385, "base path"=w3386, "file index"=w3387, "data column"="timi", "data"=w3395) -> ()  [unwired: 7 out]
                          n1484 = call "writebinary.vi"(7:w3385, "base path"=w3386, "file index"=w3387, "data column"="bdti", "data"=w3394) -> ()  [unwired: 7 out]
                          n1485 = call "writebinary.vi"(7:w3385, "base path"=w3386, "file index"=w3387, "data column"="bcli", "data"=w3393) -> ()  [unwired: 7 out]
                        }
                        frame 1 {
                          n1486 = call "writebinary.vi"(7:w3396, "base path"=w3401, "file index"=w3402, "data column"="dati", "data"=w3397) -> ()  [unwired: 7 out]
                          n1487 = call "writebinary.vi"(7:w3396, "base path"=w3401, "file index"=w3402, "data column"="timi", "data"=w3400) -> ()  [unwired: 7 out]
                          n1488 = call "writebinary.vi"(7:w3396, "base path"=w3401, "file index"=w3402, "data column"="bdti", "data"=w3399) -> ()  [unwired: 7 out]
                          n1489 = call "writebinary.vi"(7:w3396, "base path"=w3401, "file index"=w3402, "data column"="bcli", "data"=w3398) -> ()  [unwired: 7 out]
                        }
                        frame 2 {
                          n1490 = Add(x=w3420, y=w3419) -> (x+y=w3417:dbl[])
                          n1491 = Add(x=w3424, y=w3425) -> (x+y=w3423:dbl[])
                          n1492 = Add(x=w3415, y=w3414) -> (x+y=w3413:dbl[])
                          n1493 = Add(x=w3410, y=w3409) -> (x+y=w3408:dbl[])
                          n1494 = Divide(x=w3417, y=2) -> (x/y=w3416:dbl[])
                          n1495 = Divide(x=w3413, y=2) -> (x/y=w3411:dbl[])
                          n1496 = Divide(x=w3423, y=2) -> (x/y=w3421:dbl[])
                          n1497 = call "writebinary.vi"(7:w3407, "base path"=w3426, "file index"=w3427, "data column"="dati", "data"=w3408) -> ()  [unwired: 7 out]
                          n1498 = call "writebinary.vi"(7:w3407, "base path"=w3426, "file index"=w3427, "data column"="timi", "data"=w3421) -> ()  [unwired: 7 out]
                          n1499 = call "writebinary.vi"(7:w3407, "base path"=w3426, "file index"=w3427, "data column"="bdti", "data"=w3416) -> ()  [unwired: 7 out]
                          n1500 = call "writebinary.vi"(7:w3407, "base path"=w3426, "file index"=w3427, "data column"="bcli", "data"=w3411) -> ()  [unwired: 7 out]
                        }
                        frame 3 {
                          n1501 = Add(x=w3445, y=w3444) -> (x+y=w3442:dbl[])
                          n1502 = Add(x=w3449, y=w3450) -> (x+y=w3448:dbl[])
                          n1503 = Add(x=w3440, y=w3439) -> (x+y=w3438:dbl[])
                          n1504 = Subtract(x=w3435, y=w3434) -> (x-y=w3433:dbl[])
                          n1505 = Divide(x=w3442, y=2) -> (x/y=w3441:dbl[])
                          n1506 = Divide(x=w3438, y=2) -> (x/y=w3436:dbl[])
                          n1507 = Divide(x=w3448, y=2) -> (x/y=w3446:dbl[])
                          n1508 = call "writebinary.vi"(7:w3432, "base path"=w3451, "file index"=w3452, "data column"="dati", "data"=w3433) -> ()  [unwired: 7 out]
                          n1509 = call "writebinary.vi"(7:w3432, "base path"=w3451, "file index"=w3452, "data column"="timi", "data"=w3446) -> ()  [unwired: 7 out]
                          n1510 = call "writebinary.vi"(7:w3432, "base path"=w3451, "file index"=w3452, "data column"="bdti", "data"=w3441) -> ()  [unwired: 7 out]
                          n1511 = call "writebinary.vi"(7:w3432, "base path"=w3451, "file index"=w3452, "data column"="bcli", "data"=w3436) -> ()  [unwired: 7 out]
                        }
                        frame 4 {
                          n1512 = Add(x=w3470, y=w3469) -> (x+y=w3467:dbl[])
                          n1513 = Add(x=w3474, y=w3475) -> (x+y=w3473:dbl[])
                          n1514 = Add(x=w3465, y=w3464) -> (x+y=w3463:dbl[])
                          n1515 = Subtract(x=w3459, y=w3458) -> (x-y=w3460:dbl[])
                          n1516 = Divide(x=w3467, y=2) -> (x/y=w3466:dbl[])
                          n1517 = Divide(x=w3463, y=2) -> (x/y=w3461:dbl[])
                          n1518 = Divide(x=w3473, y=2) -> (x/y=w3471:dbl[])
                          n1519 = call "writebinary.vi"(7:w3457, "base path"=w3476, "file index"=w3477, "data column"="dati", "data"=w3460) -> ()  [unwired: 7 out]
                          n1520 = call "writebinary.vi"(7:w3457, "base path"=w3476, "file index"=w3477, "data column"="timi", "data"=w3471) -> ()  [unwired: 7 out]
                          n1521 = call "writebinary.vi"(7:w3457, "base path"=w3476, "file index"=w3477, "data column"="bdti", "data"=w3466) -> ()  [unwired: 7 out]
                          n1522 = call "writebinary.vi"(7:w3457, "base path"=w3476, "file index"=w3477, "data column"="bcli", "data"=w3461) -> ()  [unwired: 7 out]
                        }
                        frame 5 {
                          n1523 = case shown="False" w3495 {
                            tunnel: w3494 -> [_ w3509]
                            tunnel: w3493 -> [w3505 _]
                            tunnel: w3492 -> [_ w3508]
                            tunnel: w3491 -> [w3504 _]
                            tunnel: w3490 -> [_ w3507]
                            tunnel: w3489 -> [w3503 _]
                            tunnel: w3488 -> [_ w3506]
                            tunnel: w3487 -> [w3502 _]
                            tunnel: [w3505 w3509] -> w3486
                            tunnel: [w3504 w3508] -> w3485
                            tunnel: [w3503 w3507] -> w3484
                            tunnel: [w3502 w3506] -> w3483
                            frame False {
                            }
                            frame True {
                            }
                          }
                          n1524 = call "writebinary.vi"(7:w3482, "base path"=w3496, "file index"=w3497, "data column"="dati", "data"=w3483) -> ()  [unwired: 7 out]
                          n1525 = call "writebinary.vi"(7:w3482, "base path"=w3496, "file index"=w3497, "data column"="timi", "data"=w3486) -> ()  [unwired: 7 out]
                          n1526 = call "writebinary.vi"(7:w3482, "base path"=w3496, "file index"=w3497, "data column"="bdti", "data"=w3485) -> ()  [unwired: 7 out]
                          n1527 = call "writebinary.vi"(7:w3482, "base path"=w3496, "file index"=w3497, "data column"="bcli", "data"=w3484) -> ()  [unwired: 7 out]
                        }
                      }
                    }
                  }
                  frame #3 {
                    n1528 = Build Array(w3795) -> (w3794:u16[])
                    n1529 = call "writebinary.vi"("base path"=w3793, "file index"=0, "data column"="inte", "data"=w3794) -> ()  [unwired: 1 in, 7 out]
                    n1530 = for {
                      tunnel: w3793 -> [w3803]
                      tunnel: w3796 -> [_] mode=indexing
                      tunnel: w3790 -> [w3797]
                      i -> [w3802]
                      n1531 = call "readbinary.vi"(7:w3797, "base path"=w3803, "file index"=w3802, "data column"="dati") -> ("data"=w3800:ext[])  [unwired: 7 out]
                      n1532 = Multiply(x=0, y=w3800) -> (x*y=w3799:ext[])
                      n1533 = call "writebinary.vi"(7:w3797, "base path"=w3803, "file index"=w3802, "data column"="temp", "data"=w3799) -> ()  [unwired: 7 out]
                    }
                    "interpolate in:" <- w3795
                  }
                  frame #4 {
                    (unwired) "dati"
                    (unwired) "bdti"
                    (unwired) "timi"
                    n1534 = for {
                      tunnel: "special background/filter operations" -> [w3820]
                      tunnel: "gamma" -> [w3819]
                      tunnel: "F" -> [w3818]
                      tunnel: "phase" -> [w3817]
                      tunnel: "amp" -> [w3816]
                      tunnel: w3807 -> [w3815]
                      tunnel: w3806 -> [_] mode=indexing
                      tunnel: w3805 -> [w3813]
                      i -> [w3814]
                      n1535 = case shown="0, Default" w3820 {
                        tunnel: w3819 -> [_ w3831 w3851 _ _]
                        tunnel: w3818 -> [_ w3830 w3850 _ _]
                        tunnel: w3817 -> [_ w3829 w3849 _ _]
                        tunnel: w3816 -> [_ w3828 w3848 _ _]
                        tunnel: w3815 -> [_ w3823 w3841 w3862 w3898]
                        tunnel: w3814 -> [_ w3824 w3842 w3863 w3899]
                        tunnel: w3813 -> [_ w3821 w3840 w3861 w3896]
                        frame 0, Default {
                        }
                        frame 1 {
                          n1536 = call "readbinary.vi"(7:w3821, "base path"=w3823, "file index"=w3824, "data column"="bcli") -> ("data"=w3826:ext[])  [unwired: 7 out]
                          n1537 = Divide(x=w3830, y=w3826) -> (x/y=w3837:ext[])
